vi "Ack_comando_arduino.vi"(8 "error in (no error)":errorcluster, 10 "?":T1, 11 "VISA resource name":refnum<visa-resource-name>) -> (0 "error IO":errorcluster, 3 "VISA resource name 2":refnum<visa-resource-name>, 4 "Movimiento realizado?":bool)   [LabVIEW 2019]
uses:
  Typedefs/Comandos.ctl
  <vilib>/Utility/error.llb/Error Cluster From Error Code.vi
  <vilib>/ErrorRing/Error Ring.xnode
panel:
  out "read buffer":string
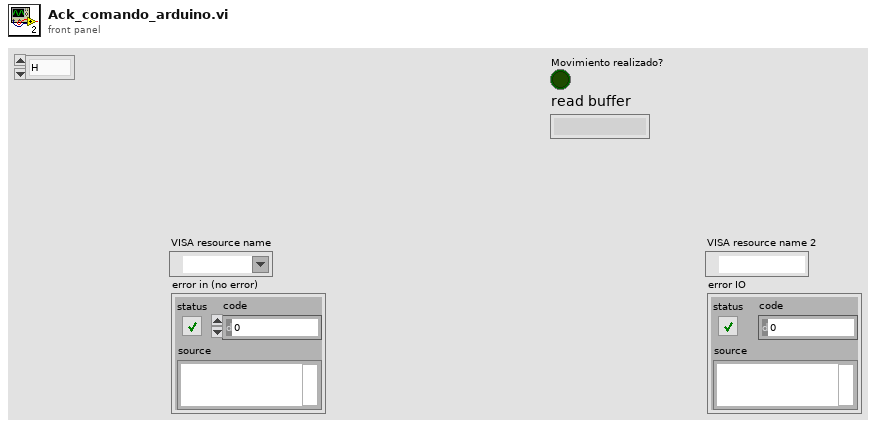
[diagram p1: front panel]
types:
  T1 = typedef "Comandos.ctl" = enum16{"H", "FH", "FM", "FI", "FX", "FY", "FZ", "I", "OK"}
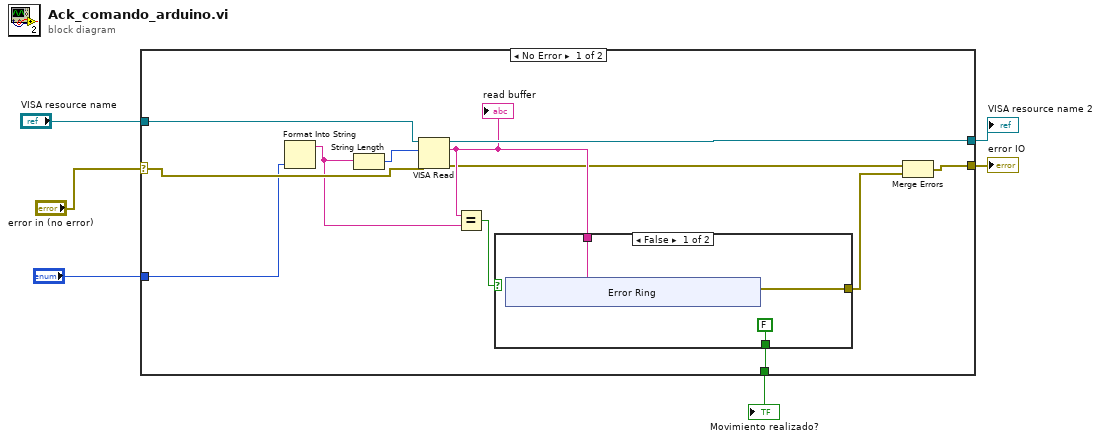
[diagram p0: block diagram]
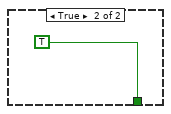
[diagram p2: hidden frame]
diagram:
  n1 = case shown="No Error" "error in (no error)" {
    selector: "error in (no error)" -> [w17 w31]
    tunnel: [w9 w31] -> w3
    tunnel: "VISA resource name" -> [w16 w30]
    tunnel: [w15 w30] -> w4
    tunnel: "?" -> [w8 _]
    tunnel: [w7 _] -> w1
    frame No Error {
      n2 = Format Into String(w8) -> (resulting string=w13:string)  [unwired: 3 in, 1 out]
      n3 = String Length(string=w13) -> (length=w18:i32)
      n4 = VISA Read(VISA resource name=w16, byte count=w18, error in (no error)=w17) -> (VISA resource name out=w15:refnum<visa-resource-name>, read buffer=w12:string, error out=w10:errorcluster)  [unwired: 1 out]
      "read buffer" <- w12
      n5 = Equal?(x=w12, y=w13) -> (x = y?=w14:bool)
      n6 = case shown="False" w14 {
        tunnel: w12 -> [w21 _]
        tunnel: [w20 _] -> w11
        tunnel: [FALSE TRUE] -> w7
        frame False {
          n7 = xnode "Error Ring"("parameter 0"=w21) -> ("error out"=w20:errorcluster)
        }
        frame True {
        }
      }
      n8 = Merge Errors(w10, w11) -> (w9:errorcluster)
    }
    frame Error {
    }
  }
  "VISA resource name 2" <- w4
  "error IO" <- w3
  "Movimiento realizado?" <- w1
